vi "DoesScriptExist.vi"(11 "File Name With Extension":string) -> (2 "file or folder exists?":bool)   [LabVIEW 2015]
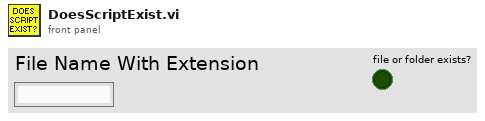
[diagram p1: front panel]
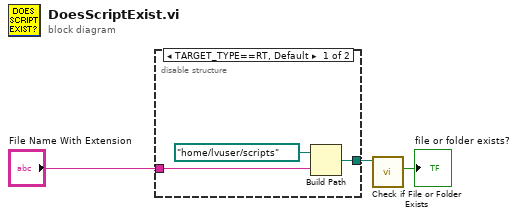
[diagram p0: block diagram]
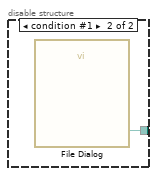
[diagram p2: hidden frame]
diagram:
  n1 = disable-structure shown="TARGET_TYPE==RT, Default" {
    disable-tunnel: "File Name With Extension" -> [w6 _]
    disable-tunnel: [w4 w7] -> w1
    frame condition #0 (active) {
      n2 = Build Path(base path=path "/home/lvuser/scripts", name or relative path=w6) -> (appended path=w4:path)
    }
    frame condition #1 {
      n3 = call "File Dialog"() -> ("selected path"=w7:path)  [unwired: 7 in, 8 out]
    }
  }
  n4 = call <vilib>:"Check if File or Folder Exists.vi"("path"=w1) -> ("file or folder exists?"=→"file or folder exists?":bool)  [unwired: 1 in, 9 out]
